vi "Test Read Date & Time.vi"(11 "TwinCAT ADS in":refnum<class "TwinCAT ADS.lvclass">) -> (3 "TwinCAT ADS out":refnum<class "TwinCAT ADS.lvclass">)   [LabVIEW 2018]
uses:
  TwinCAT ADS Class/TwinCAT ADS.lvclass
  e6b7c237-0404-4c2a-81ac-483b176eb2c7.vi
  248ffe81-f972-488d-b707-bf2a1fe23b26.vi
  0e239156-c8b5-4e08-92aa-d416179bb76f.vi
  da5912db-239c-466c-8894-2e4d3d3515d5.vi
  0b8e16e0-dc07-46b7-b0c9-e61de058ac04.vi
  9020aa95-6034-4dbf-83dd-b9edd1e76234.vi
  e5c40106-6d15-478c-83d1-da726149c43f.vi
  d432d6b6-cb13-4d15-9f79-374da6932203.vi
  66708433-c380-4caa-81db-290be98b0d9d.vi
  0e82c4fa-873b-4361-ac99-2e6e4b7cd392.vi
  da0f88be-82f8-4e5b-86e7-5baa69d9b51e.vi
  4782b519-43e7-4b8e-bd72-e209be860882.vi
  e7a7b24b-aede-49d7-b369-bb451e1de87e.vi
  TwinCAT ADS Class/VIs/Data/Read.vi
  <vilib>/addons/_JKI Toolkits/Caraya/classes/Assert/Assert Equal Value and Type_Variant.vi
  <vilib>/addons/_JKI Toolkits/Caraya/classes/Assert/Assert.lvclass
  <vilib>/addons/_JKI Toolkits/Caraya/classes/Test/Test.lvclass
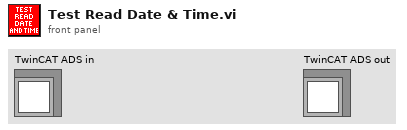
[diagram p1: front panel]
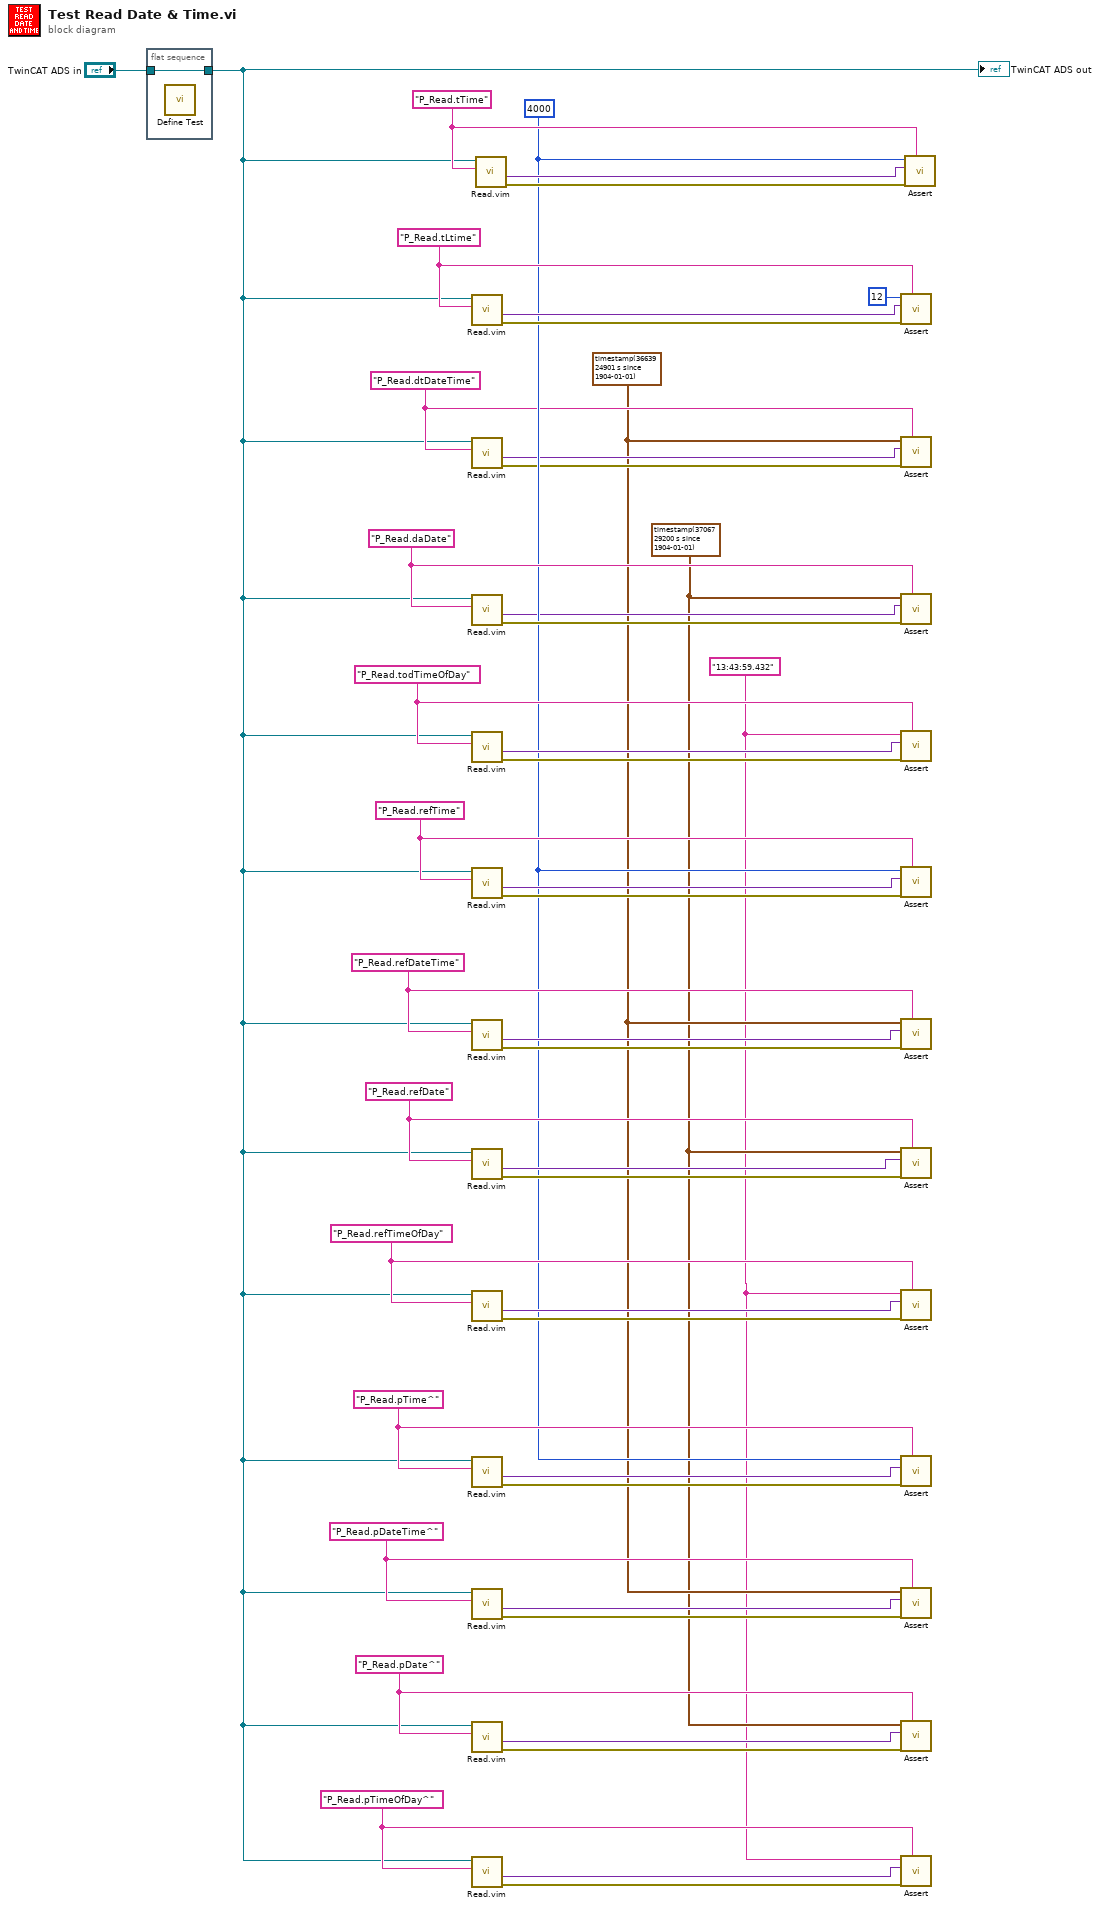
[diagram p0: block diagram]
diagram:
  w2 = timestamp(3706729200 s since 1904-01-01) ("Value")
  w6 = "P_Read.dtDateTime" ("Symbol Name")
  w3 = timestamp(3663924901 s since 1904-01-01) ("Value")
  w9 = u32 4000
  w13 = "P_Read.pTimeOfDay^" ("Symbol Name")
  w14 = "P_Read.pDate^" ("Symbol Name")
  w19 = "P_Read.pDateTime^" ("Symbol Name")
  w20 = "P_Read.pTime^" ("Symbol Name")
  w1 = "13:43:59.432" ("Symbol Name")
  w29 = "P_Read.refTimeOfDay" ("Symbol Name")
  w30 = "P_Read.refDate" ("Symbol Name")
  w33 = "P_Read.refDateTime" ("Symbol Name")
  w34 = "P_Read.refTime" ("Symbol Name")
  w39 = "P_Read.todTimeOfDay" ("Symbol Name")
  w40 = "P_Read.daDate" ("Symbol Name")
  w43 = "P_Read.tLtime" ("Symbol Name")
  w44 = "P_Read.tTime" ("Symbol Name")
  n1 = flat-sequence {
    tunnel: "TwinCAT ADS in" -> [w47]
    tunnel: [w47] -> w5
    frame #0 {
      n2 = call <vilib>:"Define Test.vi"() -> ()  [unwired: 10 in, 2 out]
    }
  }
  n3 = call "Read.vim"("Symbol Name"=w43, "TwinCAT ADS in"=w5) -> ("error out"=w42:errorcluster, "Value"=w36:variant)  [unwired: 7 in, 1 out]
  n4 = call "Read.vim"("Symbol Name"=w6, "TwinCAT ADS in"=w5) -> ("error out"=w7:errorcluster, "Value"=w8:variant)  [unwired: 7 in, 1 out]
  n5 = call "Read.vim"("Symbol Name"=w40, "TwinCAT ADS in"=w5) -> ("error out"=w41:errorcluster, "Value"=w4:variant)  [unwired: 7 in, 1 out]
  n6 = call "Read.vim"("Symbol Name"=w39, "TwinCAT ADS in"=w5) -> ("error out"=w38:errorcluster, "Value"=w26:variant)  [unwired: 7 in, 1 out]
  n7 = call "Read.vim"("Symbol Name"=w34, "TwinCAT ADS in"=w5) -> ("error out"=w35:errorcluster, "Value"=w27:variant)  [unwired: 7 in, 1 out]
  n8 = call "Read.vim"("Symbol Name"=w33, "TwinCAT ADS in"=w5) -> ("error out"=w32:errorcluster, "Value"=w25:variant)  [unwired: 7 in, 1 out]
  n9 = call "Read.vim"("Symbol Name"=w30, "TwinCAT ADS in"=w5) -> ("error out"=w31:errorcluster, "Value"=w24:variant)  [unwired: 7 in, 1 out]
  n10 = call "Read.vim"("Symbol Name"=w29, "TwinCAT ADS in"=w5) -> ("error out"=w28:errorcluster, "Value"=w23:variant)  [unwired: 7 in, 1 out]
  n11 = call "Read.vim"("Symbol Name"=w20, "TwinCAT ADS in"=w5) -> ("error out"=w21:errorcluster, "Value"=w22:variant)  [unwired: 7 in, 1 out]
  n12 = call "Read.vim"("Symbol Name"=w19, "TwinCAT ADS in"=w5) -> ("error out"=w18:errorcluster, "Value"=w17:variant)  [unwired: 7 in, 1 out]
  n13 = call "Read.vim"("Symbol Name"=w14, "TwinCAT ADS in"=w5) -> ("error out"=w15:errorcluster, "Value"=w16:variant)  [unwired: 7 in, 1 out]
  n14 = call "Read.vim"("Symbol Name"=w13, "TwinCAT ADS in"=w5) -> ("error out"=w12:errorcluster, "Value"=w11:variant)  [unwired: 7 in, 1 out]
  n15 = call "Read.vim"("Symbol Name"=w44, "TwinCAT ADS in"=w5) -> ("error out"=w46:errorcluster, "Value"=w37:variant)  [unwired: 7 in, 1 out]
  n16 = call-poly <vilib>:"Assert.vi"("Label"=w43, "error in (no error)"=w42, "Y"=w36, "X"=u64 12) -> ()  [unwired: 6 in, 2 out]
  n17 = call-poly <vilib>:"Assert.vi"("Label"=w6, "error in (no error)"=w7, "Y"=w8, "X"=w3) -> ()  [unwired: 6 in, 2 out]
  n18 = call-poly <vilib>:"Assert.vi"("Label"=w40, "error in (no error)"=w41, "Y"=w4, "X"=w2) -> ()  [unwired: 6 in, 2 out]
  n19 = call-poly <vilib>:"Assert.vi"("Label"=w39, "error in (no error)"=w38, "Y"=w26, "X"=w1) -> ()  [unwired: 6 in, 2 out]
  n20 = call-poly <vilib>:"Assert.vi"("Label"=w34, "error in (no error)"=w35, "Y"=w27, "X"=w9) -> ()  [unwired: 6 in, 2 out]
  n21 = call-poly <vilib>:"Assert.vi"("Label"=w33, "error in (no error)"=w32, "Y"=w25, "X"=w3) -> ()  [unwired: 6 in, 2 out]
  n22 = call-poly <vilib>:"Assert.vi"("Label"=w30, "error in (no error)"=w31, "Y"=w24, "X"=w2) -> ()  [unwired: 6 in, 2 out]
  n23 = call-poly <vilib>:"Assert.vi"("Label"=w29, "error in (no error)"=w28, "Y"=w23, "X"=w1) -> ()  [unwired: 6 in, 2 out]
  n24 = call-poly <vilib>:"Assert.vi"("Label"=w20, "error in (no error)"=w21, "Y"=w22, "X"=w9) -> ()  [unwired: 6 in, 2 out]
  n25 = call-poly <vilib>:"Assert.vi"("Label"=w19, "error in (no error)"=w18, "Y"=w17, "X"=w3) -> ()  [unwired: 6 in, 2 out]
  n26 = call-poly <vilib>:"Assert.vi"("Label"=w14, "error in (no error)"=w15, "Y"=w16, "X"=w2) -> ()  [unwired: 6 in, 2 out]
  n27 = call-poly <vilib>:"Assert.vi"("Label"=w13, "error in (no error)"=w12, "Y"=w11, "X"=w1) -> ()  [unwired: 6 in, 2 out]
  n28 = call-poly <vilib>:"Assert.vi"("Label"=w44, "error in (no error)"=w46, "Y"=w37, "X"=w9) -> ()  [unwired: 6 in, 2 out]
  "TwinCAT ADS out" <- w5
